vi "midi_in.device_count.get.vi"(8 "error in (no error)":errorcluster, 11 "LabVIEW-MIDI-XPLAT in":refnum<class "LabVIEW-MIDI-XPLAT.lvclass">) -> (0 "error out":errorcluster, 2 "device count":i32, 3 "LabVIEW-MIDI-XPLAT out":refnum<class "LabVIEW-MIDI-XPLAT.lvclass">)   [LabVIEW 2020, in "LabVIEW-MIDI-XPLAT.lvclass"]
uses:
  LabVIEW-MIDI-XPLAT.lvclass
  target/release/midi_driver.dll
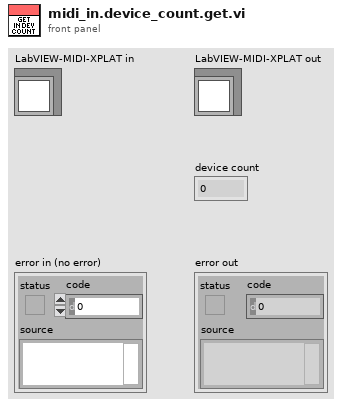
[diagram p1: front panel]
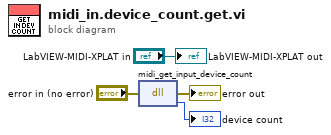
[diagram p0: block diagram]
diagram:
  n1 = dll-call lib="C:/code/LabVIEW-MIDI-XPLAT/target/release/midi_driver.dll" fn="midi_get_input_device_count"(error in="error in (no error)") -> (error out=→"error out":errorcluster, "device count"=→"device count":i32)  [unwired: 2 in, 1 out]
  "LabVIEW-MIDI-XPLAT out" <- "LabVIEW-MIDI-XPLAT in"
